vi "Write Player Info.vi"(8 "error in (no error)":errorcluster, 10 "Player Info":T1={"Name"="", "Color Box"=0, "Gloat Phrase"="All your base are belong to us!!"}, 11 "Scout in":refnum<class "Scout.lvclass">) -> (0 "error out":errorcluster, 3 "Scout out":refnum<class "Scout.lvclass">)   [LabVIEW 2014, in "Scout.lvclass"]
uses:
  Scout.lvclass
  Player Info.ctl
  Formics/Formics.lvclass
  SquareBattle Arena/SquareBattle Arena.lvclass
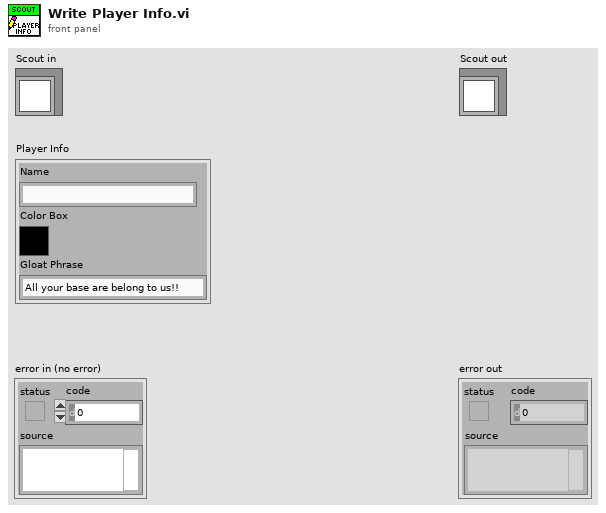
[diagram p1: front panel]
types:
  T1 = typedef "SquareBattle Arena.lvlib/SquareBattle Arena.lvclass/Player Info.ctl" = cluster{"Name":string, "Color Box":u32, "Gloat Phrase":string}
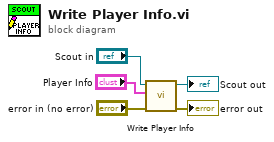
[diagram p0: block diagram]
diagram:
  n1 = call-parent "Write Player Info.vi"("error in (no error)"="error in (no error)", "Player Info"="Player Info", "Mother in"="Scout in") -> ("error out"=→"error out":errorcluster, "Mother out"=→"Scout out":refnum<class "Scout.lvclass">)  [unwired: 7 in]
